vi "GetDisplayBounds.vi"(8 "No Error":errorcluster, 11 "Display ID":T2) -> (0 "Error Out":errorcluster, 3 "Rect":T1)   [LabVIEW 2026, in "SDL3.lvlib" / "Video.lvlib"]
doc: "<B>Summary</B>\nGet the desktop area represented by a display.\n\n<B>Remarks</B>\nThe primary display is always located at (0,0)."
uses:
  Video.lvlib
  DisplayID--integer.ctl
  Rect/Rect--cluster.ctl
  <vilib>/Utility/error.llb/Error Cluster From Error Code.vi
  Rect/Rect.lvlib
  Error/Error.lvlib
  Lib/SDL3.dll
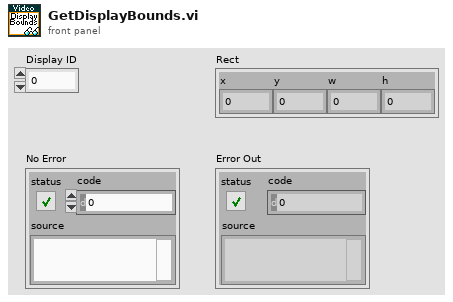
[diagram p1: front panel]
types:
  T1 = typedef "SDL3.lvlib/Rect.lvlib/Rect--cluster.ctl" = cluster{"x":i32, "y":i32, "w":i32, "h":i32}
  T2 = typedef "SDL3.lvlib/Video.lvlib/DisplayID--integer.ctl" = u32
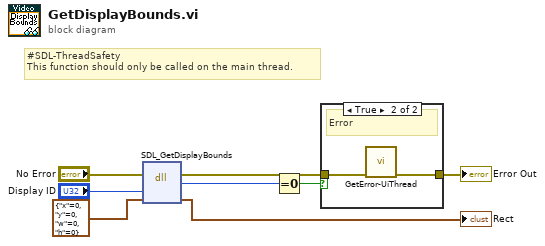
[diagram p0: block diagram]
diagram:
  # "#SDL-ThreadSafety\nThis function should only be called on the main thread."
  n1 = dll-call lib="C:/Users/saukko/Dev/LV-SDL3/Sources/SDL3/Lib/SDL3.*" fn="SDL_GetDisplayBounds"(error in="No Error", "displayID"="Display ID", "rect"=T1 {"x"=0, "y"=0, "w"=0, "h"=0} ("Rect")) -> (error out=w4:errorcluster, "return type"=w5:i32, "rect"=→"Rect":T1)  [unwired: 3 in, 1 out]
  n2 = Equal To 0?(x=w5) -> (x = 0?=w3:bool)
  n3 = case shown="True" w3 {
    tunnel: w4 -> [w9 w11]
    tunnel: [w9 w10] -> w7
    frame False {
      # "Ok"
    }
    frame True {
      # "Error"
      n4 = call "GetError-UiThread.vi"("No Error"=w11) -> ("error out"=w10:errorcluster)  [unwired: 10 in]
    }
  }
  "Error Out" <- w7
